vi "Message Packet Encoding.vi"(8 "error in (no error)":errorcluster, 10 "Message Packet In":T1, 11 "HSMS Class in":refnum<class "HSMS Class.lvclass">) -> (0 "error out":errorcluster, 1 "Data":string, 2 "Message Packet Out":T1, 3 "HSMS Class out":refnum<class "HSMS Class.lvclass">)   [LabVIEW 2020, in "SECS Communication.lvlib" / "HSMS Class.lvclass"]
uses:
  HSMS Class.lvclass
  Message Packet.ctl
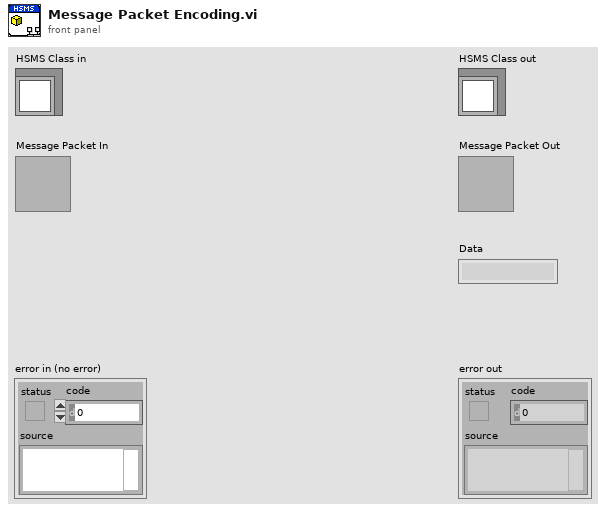
[diagram p1: front panel]
types:
  T1 = typedef "SECS Communication.lvlib/HSMS Class.lvclass/Message Packet.ctl" = cluster{"Message Header Cluster":T2, "Message Header":u8[], "Message Text":u8[]}
  T2 = typedef "SECS Communication.lvlib/HSMS Class.lvclass/Message Header.ctl" = cluster{"Byte 0-1(Session ID)":u16, "W-Bit":bool, "Byte 2":u8, "Byte 3":u8, "Byte 4(PType)":T3, "Byte 5(SType)":T4, "Byte 6-9(System Btyes)":u8[]}
  T3 = typedef "SECS Communication.lvlib/HSMS Class.lvclass/PType.ctl" = enum8{"SECS-II Encoding", "Reserved"}
  T4 = typedef "SECS Communication.lvlib/HSMS Class.lvclass/SType.ctl" = enum8{"Data Message", "Select.req", "Select.rsp", "Deselect.req", "Deselect.rsp", "Linktest.req", "Linktest.rsp", "Reject.req", "Separate.req"}
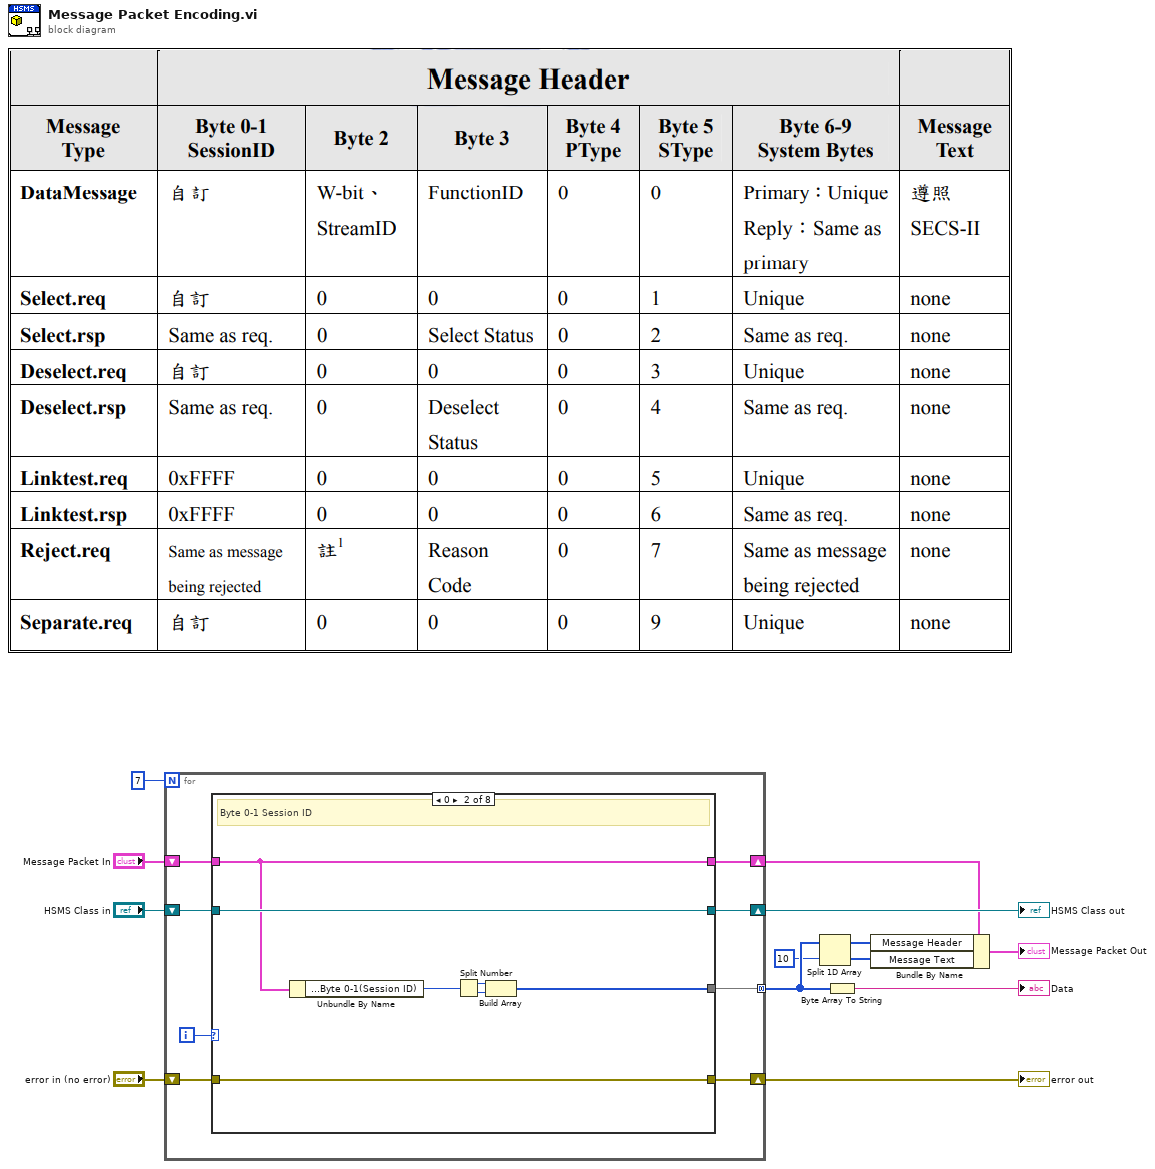
[diagram p0: block diagram]
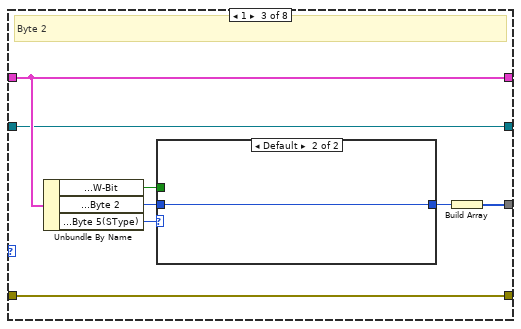
[diagram p3: hidden frame]
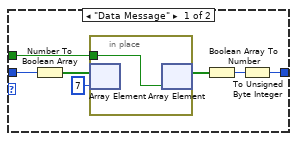
[diagram p4: hidden frame]
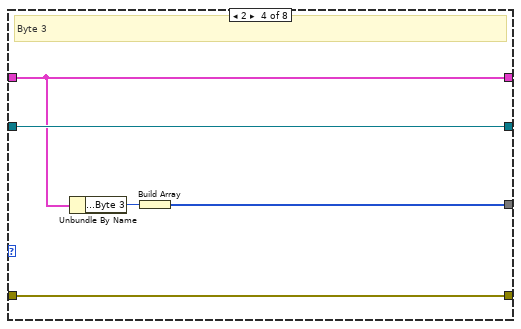
[diagram p5: hidden frame]
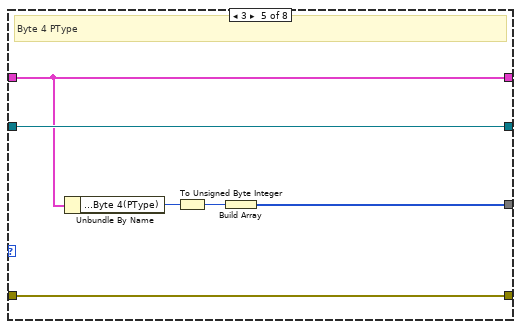
[diagram p6: hidden frame]
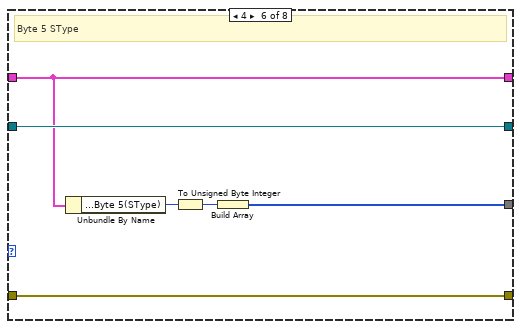
[diagram p7: hidden frame]
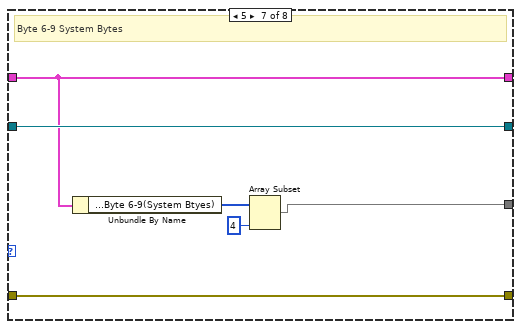
[diagram p8: hidden frame]
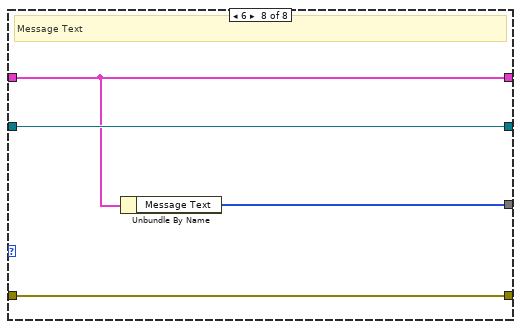
[diagram p9: hidden frame]
diagram:
  n1 = for {
    N: 7 -> [_]
    tunnel: [w18] -> w6 mode=concatenating
    shift-right: [w16] -> w10
    shift-left: "error in (no error)" -> [w20]
    shift-right: [w14] -> w4
    shift-left: "Message Packet In" -> [w15]
    shift-right: [w17] -> w9
    shift-left: "HSMS Class in" -> [w19]
    i -> [w21]
    n2 = case shown="0" w21 {
      tunnel: w20 -> [w23 w27 w32 w52 w56 w62 w70 w73]
      tunnel: w19 -> [w24 w28 w35 w51 w55 w61 w71 w74]
      tunnel: [_ w31 w37 w53 w57 w63 w68 w75] -> w18
      tunnel: [w24 w28 w35 w51 w55 w61 w71 w74] -> w17
      tunnel: [w23 w27 w32 w52 w56 w62 w70 w73] -> w16
      tunnel: w15 -> [w22 w26 w36 w49 w54 w60 w66 w72]
      tunnel: [w22 w26 w36 w49 w54 w60 w66 w72] -> w14
      frame Default {
      }
      frame 0 {
        # "Byte 0-1 Session ID"
        n3 = Unbundle By Name(w26) -> ("Message Header Cluster.Byte 0-1(Session ID)"=w25:u16)
        n4 = Split Number(x=w25) -> (hi(x)=w30:u8, lo(x)=w29:u8)
        n5 = Build Array(w30, w29) -> (w31:u8[])
      }
      frame 1 {
        # "Byte 2"
        n6 = Unbundle By Name(w36) -> ("Message Header Cluster.W-Bit"=w33:bool, "Message Header Cluster.Byte 2"=w34:u8, "Message Header Cluster.Byte 5(SType)"=w39:T4)
        n7 = case shown="Default" w39 {
          tunnel: [w42 w48] -> w38
          tunnel: w34 -> [w40 w48]
          tunnel: w33 -> [w41 _]
          frame "Data Message" {
            n8 = Number To Boolean Array(number=w40) -> (Boolean array=w45:bool[])
            n9 = in-place {
              in-place-border: w41 -> [w47]
              n10 = in-place-array #1(w45, 7 ("index")) -> ()  [unwired: 1 out]
              n11 = in-place-array #1(w47) -> (w43:bool[])  [unwired: 1 out]
            }
            n12 = Boolean Array To Number(Boolean array=w43) -> (number=w46:u32)
            n13 = To Unsigned Byte Integer(number=w46) -> (unsigned 8bit integer=w42:u8)
          }
          frame Default {
          }
        }
        n14 = Build Array(w38) -> (w37:u8[])
      }
      frame 2 {
        # "Byte 3"
        n15 = Unbundle By Name(w49) -> ("Message Header Cluster.Byte 3"=w50:u8)
        n16 = Build Array(w50) -> (w53:u8[])
      }
      frame 3 {
        # "Byte 4 PType"
        n17 = Unbundle By Name(w54) -> ("Message Header Cluster.Byte 4(PType)"=w59:T3)
        n18 = To Unsigned Byte Integer(number=w59) -> (unsigned 8bit integer=w58:u8)
        n19 = Build Array(w58) -> (w57:u8[])
      }
      frame 4 {
        # "Byte 5 SType"
        n20 = Unbundle By Name(w60) -> ("Message Header Cluster.Byte 5(SType)"=w65:T4)
        n21 = To Unsigned Byte Integer(number=w65) -> (unsigned 8bit integer=w64:u8)
        n22 = Build Array(w64) -> (w63:u8[])
      }
      frame 5 {
        # "Byte 6-9 System Bytes"
        n23 = Unbundle By Name(w66) -> ("Message Header Cluster.Byte 6-9(System Btyes)"=w67:u8[])
        n24 = Array Subset(array=w67, length=4) -> (w68:u8[])  [unwired: 1 in]
      }
      frame 6 {
        # "Message Text"
        n25 = Unbundle By Name(w72) -> ("Message Text"=w75:u8[])
      }
    }
  }
  "error out" <- w10
  "HSMS Class out" <- w9
  n26 = Split 1D Array(array=w6, index=10 ("length")) -> (first subarray=w3:u8[], second subarray=w2:u8[])
  n27 = Byte Array To String(unsigned byte array=w6) -> (string=→"Data":string)
  n28 = Bundle By Name(cluster=w4, "Message Header"=w3, "Message Text"=w2) -> (→"Message Packet Out":T1)
